vi "G#Object_GetAllObjectsFromSameOwner.vi"(1 "full class name (\"\")":string, 5 "error in (no error)":errorcluster) -> (12 "all refs":refnum<class "G#Object.lvclass">[](array[class]), 15 "external creator process owns":bool, 16 "no other owners":bool, 19 "error out":errorcluster)   [LabVIEW 2020, in "G#Object.lvclass"]
doc: "Returns all objects of the specified class with the same owner that called this method. If \"full class name\" is empty, all objects of all classes will be returned."
uses:
  <vilib>/addons/_AddQ/G#Object/G#Object.lvclass
  <vilib>/addons/_AddQ/G#Object/G#Object.lvclass/G#Object.ctl
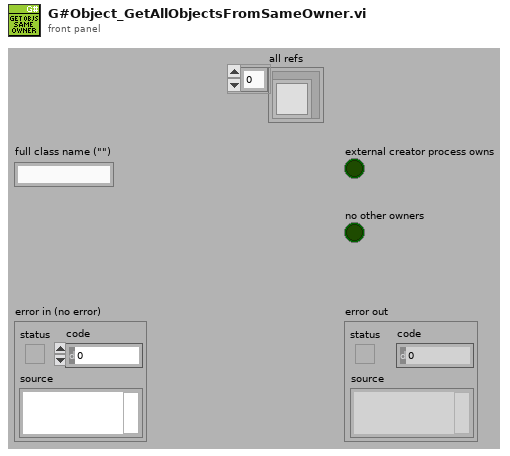
[diagram p1: front panel]
types:
  T1 = cluster{"full class name (\"\")":string, "Ref":refnum<class "G#Object.lvclass">}
  T2 = cluster{"full class name (\"\")":string, "Ref":refnum<class "G#Object.lvclass">}[]
  T3 = typedef "G#Object.lvclass/G#Object_ObjectInfoType.ctl" = cluster{"ObjectName":string, "ObjectID":u32, "Users":i32, "Counter":bool, "AttributeRefs":u32[], "FullClassName":string, "ClassName":string, "CreateMethod":T4, "GenericDestructorExists":bool, "Owner":string}
  T4 = typedef "G#Object.lvclass/G#Object_CreateMethod.ctl" = enum16{"Create", "Create or look up existing", "Look up existing"}
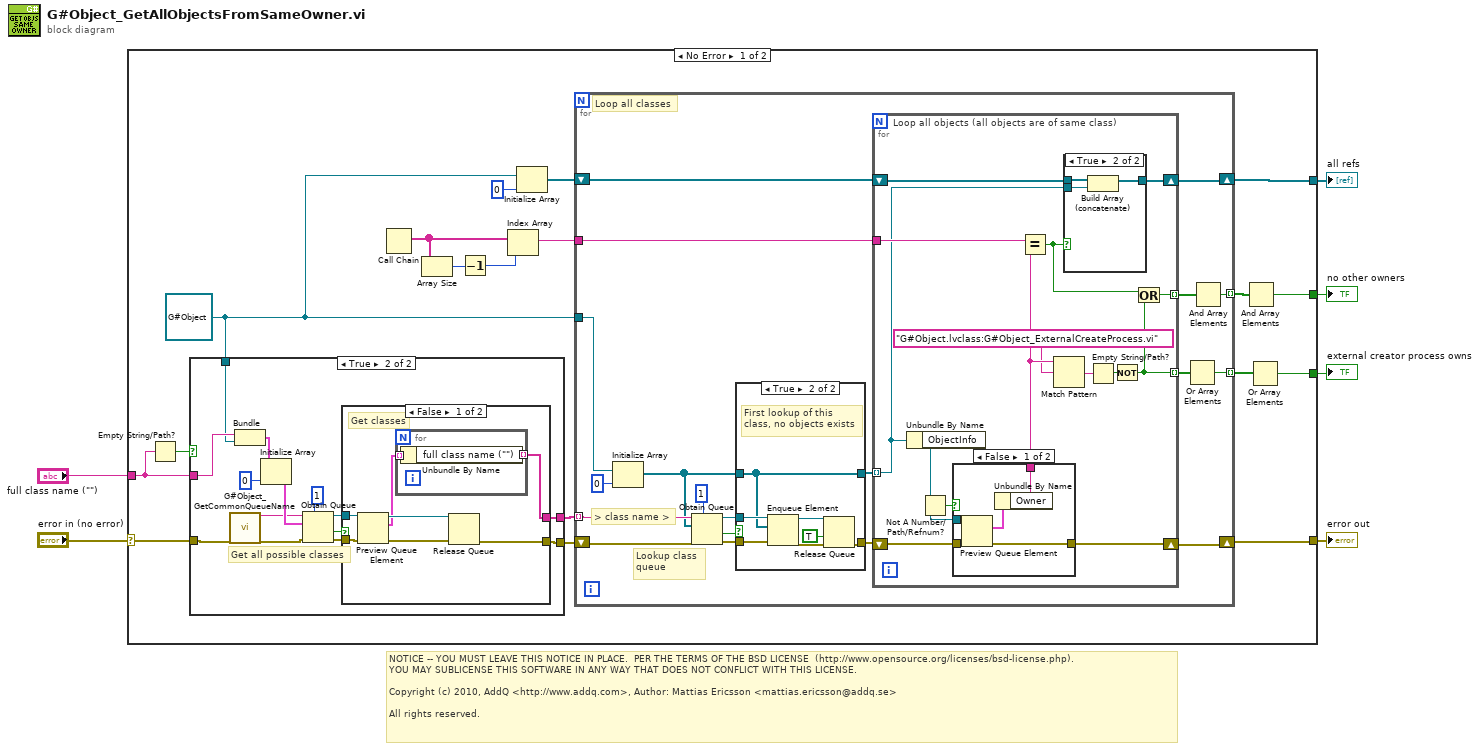
[diagram p0: block diagram]
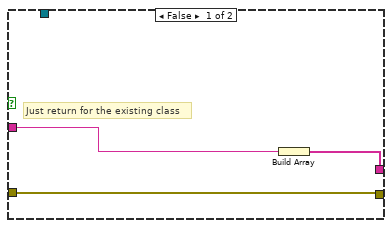
[diagram p2: hidden frame]
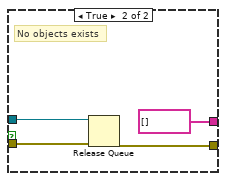
[diagram p3: hidden frame]
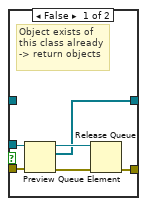
[diagram p6: hidden frame]
diagram:
  # "NOTICE -- YOU MUST LEAVE THIS NOTICE IN PLACE.  PER THE TERMS OF THE BSD LICENSE  (http://www.opensource.org/licenses/bsd-license.php).\nYOU MAY SUBLICENSE THIS SOFTWARE IN ANY WAY THAT DOES NOT CONFLICT WITH THIS LICENSE.\n\nCopyright (c) 2010, AddQ <http://www.addq.com>, Author: Mattias Ericsson <mattias.ericsson@addq.se>\n\nAll rights reserved."
  n1 = case shown="No Error" "error in (no error)" {
    selector: "error in (no error)" -> [w21 w112]
    tunnel: [w18 w112] -> w5
    tunnel: [w20 _] -> w4
    tunnel: "full class name (\"\")" -> [w16 _]
    tunnel: [w13 _] -> w2
    tunnel: [w11 _] -> w1
    frame No Error {
      w15 = refnum<class "G#Object.lvclass"> refnum ("Ref")
      n2 = Empty String/Path?(string/path=w16) -> (empty?=w17:bool)
      n3 = case shown="True" w17 {
        tunnel: [w26 w35] -> w23
        tunnel: [w27 w34] -> w22
        tunnel: w21 -> [w27 w30]
        tunnel: w16 -> [w25 w32]
        tunnel: w15 -> [_ w31]
        frame False {
          # "Just return for the existing class"
          n4 = Build Array(w25) -> (w26:string[])
        }
        frame True {
          # "Get all possible classes"
          n5 = call <vilib>:"G#Object_GetCommonQueueName.vi"("error in (no error)"=w30) -> ("queue name"=w28:string, "error out"=w29:errorcluster)  [unwired: 17 in]
          n6 = Bundle("full class name (\"\")"=w32, "Ref"=w31) -> (w33:T1)  [unwired: 1 in]
          n7 = Initialize Array(w33, 0 ("dimension size")) -> (w36:T2)
          n8 = Obtain Queue(max queue size (-1, unlimited)=1, name (unnamed)=w28, element data type=w36, error in (no error)=w29) -> (queue out=w39:refnum<queue>, created new?=w41:bool, error out=w40:errorcluster)  [unwired: 1 in]
          n9 = case shown="False" w41 {
            tunnel: w40 -> [w48 w51]
            tunnel: w39 -> [w47 w52]
            tunnel: [w43 string[] []] -> w35
            tunnel: [w46 w54] -> w34
            frame False {
              # "Get classes"
              n10 = Preview Queue Element(queue=w47, error in (no error)=w48) -> (queue out=w44:refnum<queue>, element=w42:T2, error out=w45:errorcluster)  [unwired: 1 in, 1 out]
              n11 = for {
                tunnel: [w50] -> w43 mode=indexing
                tunnel: w42 -> [w49] mode=indexing
                n12 = Unbundle By Name(w49) -> ("full class name (\"\")"=w50:string)
              }
              n13 = Release Queue(queue=w44, error in (no error)=w45) -> (error out=w46:errorcluster)  [unwired: 1 in, 2 out]
            }
            frame True {
              # "No objects exists"
              n14 = Release Queue(queue=w52, error in (no error)=w51) -> (error out=w54:errorcluster)  [unwired: 1 in, 2 out]
            }
          }
        }
      }
      n15 = Call Chain() -> (call chain=w10:string[])
      n16 = Array Size(array=w10) -> (size(s)=w9:i32)
      n17 = Decrement(x=w9) -> (x-1=w8:i32)
      n18 = Index Array(array=w10, index=w8) -> (element=w7:string)
      n19 = Initialize Array(w15, 0 ("dimension size")) -> (w24:refnum<class "G#Object.lvclass">[])
      n20 = for {
        shift-right: [w59] -> w18
        shift-left: w22 -> [w69]
        tunnel: w23 -> [w66] mode=indexing
        shift-right: [w60] -> w20
        shift-left: w24 -> [w62]
        tunnel: w15 -> [w65]
        tunnel: w7 -> [w61]
        tunnel: [w57] -> w14 mode=indexing
        tunnel: [w55] -> w12 mode=indexing
        # "Loop all classes"
        # "> class name >"
        # "Lookup class\nqueue"
        n21 = Initialize Array(w65, 0 ("dimension size")) -> (w64:refnum<class "G#Object.lvclass">[])
        n22 = Obtain Queue(max queue size (-1, unlimited)=1, name (unnamed)=w66, element data type=w64, error in (no error)=w69) -> (queue out=w70:refnum<queue>, created new?=w71:bool, error out=w72:errorcluster)  [unwired: 1 in]
        n23 = case shown="True" w71 {
          tunnel: w72 -> [w103 w111]
          tunnel: w70 -> [w102 w110]
          tunnel: w64 -> [_ w109]
          tunnel: [w104 w105] -> w68
          tunnel: [w99 w109] -> w67
          frame False {
            # "Object exists of\nthis class already\n-> return objects"
            n24 = Preview Queue Element(queue=w102, error in (no error)=w103) -> (queue out=w100:refnum<queue>, element=w99:refnum<class "G#Object.lvclass">[], error out=w101:errorcluster)  [unwired: 1 in, 1 out]
            n25 = Release Queue(queue=w100, error in (no error)=w101) -> (error out=w104:errorcluster)  [unwired: 1 in, 2 out]
          }
          frame True {
            # "First lookup of this\nclass, no objects exists"
            n26 = Enqueue Element(queue=w110, element=w109, error in (no error)=w111) -> (queue out=w107:refnum<queue>, error out=w106:errorcluster)  [unwired: 1 in, 1 out]
            n27 = Release Queue(queue=w107, force destroy? (F)=TRUE, error in (no error)=w106) -> (error out=w105:errorcluster)  [unwired: 2 out]
          }
        }
        n28 = for {
          shift-right: [w87] -> w59
          shift-left: w68 -> [w88]
          tunnel: w67 -> [w83] mode=indexing
          shift-right: [w84] -> w60
          shift-left: w62 -> [w85]
          tunnel: w61 -> [w86]
          tunnel: [w82] -> w58 mode=indexing
          tunnel: [w76] -> w56 mode=indexing
          # "Loop all objects (all objects are of same class)"
          n29 = Unbundle By Name(w83) -> ("ObjectInfo"=w75:refnum<queue>)
          n30 = Not A Number/Path/Refnum?(number/path/refnum=w75) -> (NaN/Path/Refnum?=w74:bool)
          n31 = case shown="False" w74 {
            tunnel: w88 -> [w93 w94]
            tunnel: [w92 w94] -> w87
            tunnel: [w90 _] -> w80
            tunnel: w75 -> [w89 _]
            frame False {
              n32 = Preview Queue Element(queue=w89, error in (no error)=w93) -> (element=w91:T3, error out=w92:errorcluster)  [unwired: 1 in, 2 out]
              n33 = Unbundle By Name(w91) -> ("Owner"=w90:string)
            }
            frame True {
            }
          }
          n34 = Equal?(x=w86, y=w80) -> (x = y?=w81:bool)
          n35 = Match Pattern(string=w80, regular expression="G#Object.lvclass:G#Object_ExternalCreateProcess.vi") -> (match substring=w78:string)  [unwired: 1 in, 3 out]
          n36 = case shown="True" w81 {
            tunnel: w85 -> [w95 w98]
            tunnel: [w95 w97] -> w84
            tunnel: w83 -> [_ w96]
            frame False {
            }
            frame True {
              n37 = Build Array (concatenate)(w98, w96) -> (w97:refnum<class "G#Object.lvclass">[])
            }
          }
          n38 = Empty String/Path?(string/path=w78) -> (empty?=w77:bool)
          n39 = Not(x=w77) -> (.not. x?=w76:bool)
          n40 = Or(x=w81, y=w76) -> (x .or. y?=w82:bool)
        }
        n41 = Or Array Elements(Boolean array=w56) -> (logical OR=w55:bool)
        n42 = And Array Elements(Boolean array=w58) -> (logical AND=w57:bool)
      }
      n43 = And Array Elements(Boolean array=w14) -> (logical AND=w13:bool)
      n44 = Or Array Elements(Boolean array=w12) -> (logical OR=w11:bool)
    }
    frame Error {
    }
  }
  "error out" <- w5
  "all refs" <- w4
  "no other owners" <- w2
  "external creator process owns" <- w1
